vi "Clear Steps.vi"(8 "error in (no error)":errorcluster, 11 "Sequencer in":refnum<class "Sequencer.lvclass">) -> (0 "error out":errorcluster)   [LabVIEW 2015, in "Sequencer.lvclass"]
uses:
  Sequencer.lvclass
  Sequencer.lvclass/Sequencer.ctl
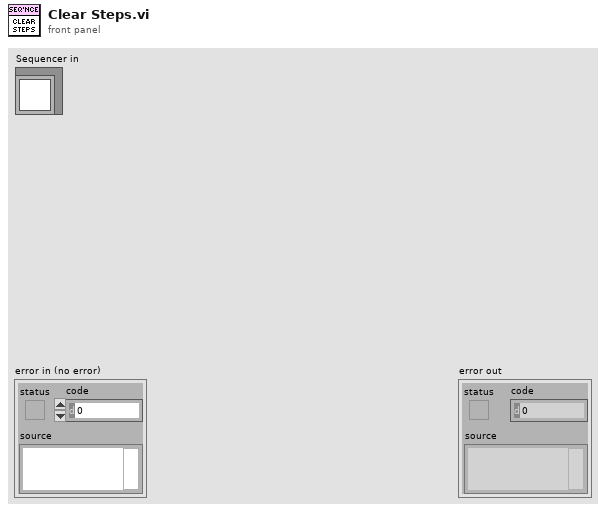
[diagram p1: front panel]
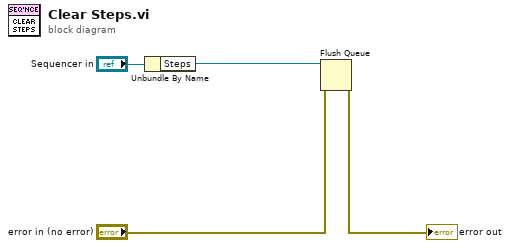
[diagram p0: block diagram]
diagram:
  n1 = Unbundle By Name("Sequencer in") -> ("Steps"=w2:refnum<queue>)
  n2 = Flush Queue(queue=w2, error in (no error)="error in (no error)") -> (error out=→"error out":errorcluster)  [unwired: 2 out]
